vi "CreateNotifier.vi"(8 "entrée d'erreur (pas d'erreur)":errorcluster) -> (0 "sortie d'erreur":errorcluster, 3 "Notifiers":T1)   [LabVIEW 2017, in "Notifier.lvlib"]
doc: "Ce VI crée tous les notifier liés à chaque appareils du centre d'usinage.\nPour l'ajout ou le retrait d'un appareil, il faut modifier ce VI.\nOn retrouve en entrée, le cluster d'erreur ; en sortie, un cluster regroupant les notifiers de chaque appareils nommer par la CTL \"notifier.ctl\", le cluster d'erreur de sortie."
uses:
  Notifier.lvlib
  Notifier.ctl
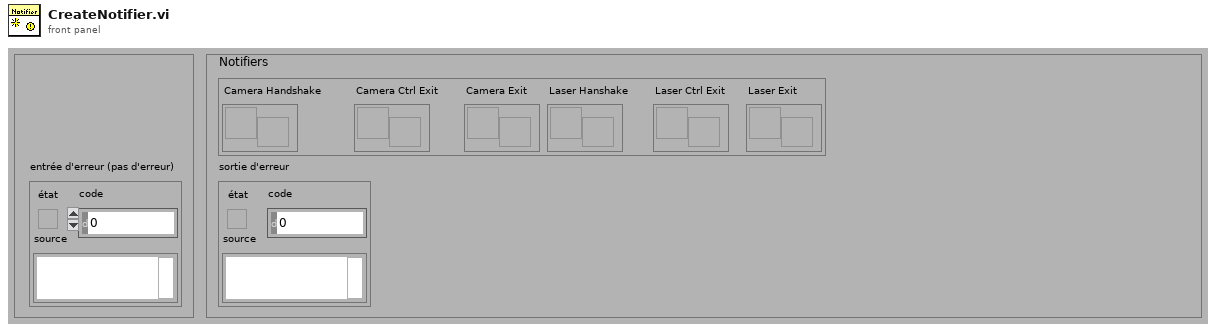
[diagram p1: front panel]
types:
  T1 = typedef "Notifier.lvlib/Notifier.ctl" = cluster{"Camera Handshake":refnum<notifier>, "Camera Ctrl Exit":refnum<notifier>, "Camera Exit":refnum<notifier>, "Laser Hanshake":refnum<notifier>, "Laser Ctrl Exit":refnum<notifier>, "Laser Exit":refnum<notifier>}
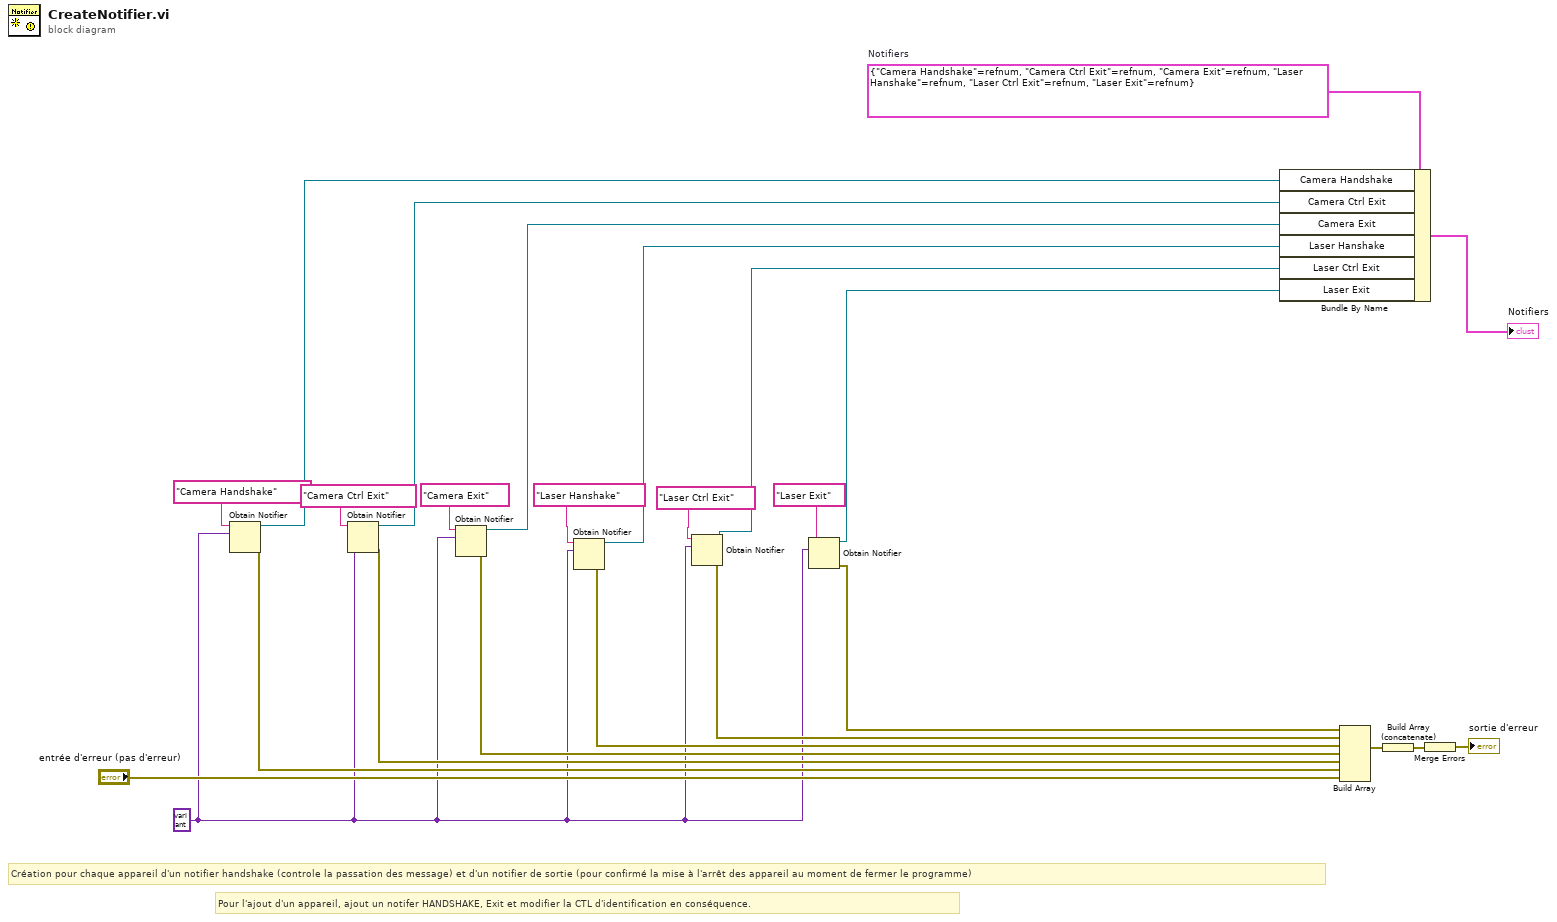
[diagram p0: block diagram]
diagram:
  w21 = T1 {"Camera Handshake"=refnum, "Camera Ctrl Exit"=refnum, "Camera Exit"=refnum, "Laser Hanshake"=refnum, "Laser Ctrl Exit"=refnum, "Laser Exit"=refnum}  # Notifiers
  w7 = variant ("variant")
  # "Pour l'ajout d'un appareil, ajout un notifer HANDSHAKE, Exit et modifier la CTL d'identification en conséquence."
  # "Création pour chaque appareil d'un notifier handshake (controle la passation des message) et d'un notifier de sortie (pour confirmé la mise à l'arrêt des appareil au moment de fermer le programme)"
  n1 = Obtain Notifier(name (unnamed)="Camera Handshake" ("nom (aucun)"), notification data type=w7) -> (notifier out=w6:refnum<notifier>, error out=w24:errorcluster)  [unwired: 2 in, 1 out]
  n2 = Obtain Notifier(name (unnamed)="Camera Ctrl Exit" ("nom (aucun)"), notification data type=w7) -> (notifier out=w1:refnum<notifier>, error out=w19:errorcluster)  [unwired: 2 in, 1 out]
  n3 = Obtain Notifier(name (unnamed)="Camera Exit" ("nom (aucun)"), notification data type=w7) -> (notifier out=w2:refnum<notifier>, error out=w18:errorcluster)  [unwired: 2 in, 1 out]
  n4 = Obtain Notifier(name (unnamed)="Laser Hanshake" ("nom (aucun)"), notification data type=w7) -> (notifier out=w3:refnum<notifier>, error out=w17:errorcluster)  [unwired: 2 in, 1 out]
  n5 = Obtain Notifier(name (unnamed)="Laser Ctrl Exit" ("nom (aucun)"), notification data type=w7) -> (notifier out=w4:refnum<notifier>, error out=w16:errorcluster)  [unwired: 2 in, 1 out]
  n6 = Obtain Notifier(name (unnamed)="Laser Exit" ("nom (aucun)"), notification data type=w7) -> (notifier out=w5:refnum<notifier>, error out=w15:errorcluster)  [unwired: 2 in, 1 out]
  n7 = Bundle By Name(cluster=w21, "Camera Handshake"=w6, "Camera Ctrl Exit"=w1, "Camera Exit"=w2, "Laser Hanshake"=w3, "Laser Ctrl Exit"=w4, "Laser Exit"=w5) -> (→"Notifiers":T1)
  n8 = Build Array(w15, w16, w17, w18, w19, w24, "entrée d'erreur (pas d'erreur)") -> (w25:errorcluster[])
  n9 = Build Array (concatenate)(w25) -> (w20:errorcluster[])
  n10 = Merge Errors(w20) -> (→"sortie d'erreur":errorcluster)
